vi "Read VI Refnum.vi"(8 "error in (no error)":errorcluster, 11 "BD_CAFE_USD_ING in":refnum<class "BD_CAFE_USD_ING.lvclass">) -> (0 "error out":errorcluster, 2 "VI Refnum":refnum<vi>, 3 "BD_CAFE_USD_ING out":refnum<class "BD_CAFE_USD_ING.lvclass">)   [LabVIEW 2019, in "BD_CAFE_USD_ING.lvlib" / "BD_CAFE_USD_ING.lvclass"]
uses:
  BD_CAFE_USD_ING.lvclass
  BD_CAFE_USD_ING.lvclass/BD_CAFE_USD_ING.ctl
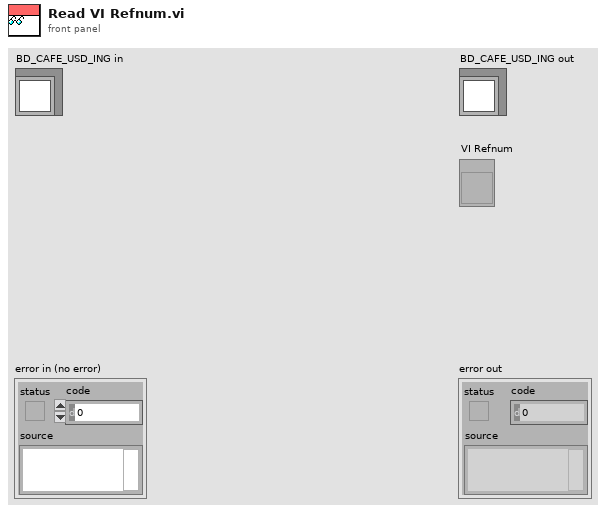
[diagram p1: front panel]
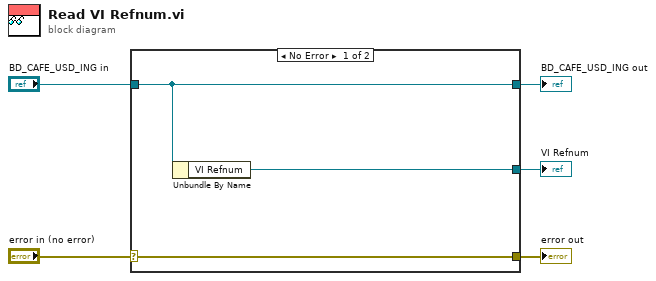
[diagram p0: block diagram]
diagram:
  n1 = case shown="No Error" "error in (no error)" {
    selector: "error in (no error)" -> [w8 w9]
    tunnel: [w8 w9] -> w4
    tunnel: [w7 w10] -> w2
    tunnel: "BD_CAFE_USD_ING in" -> [w7 w10]
    tunnel: [w6 _] -> w1
    frame No Error {
      n2 = Unbundle By Name(w7) -> ("VI Refnum"=w6:refnum<vi>)
    }
    frame Error {
    }
  }
  "error out" <- w4
  "BD_CAFE_USD_ING out" <- w2
  "VI Refnum" <- w1
